vi "Do.vi"(8 "error in (no error)":errorcluster, 10 "Actor in":refnum<class "Actor.lvclass">, 11 "Configure Ports Msg":refnum<class "Configure Ports Msg.lvclass">) -> (0 "error out":errorcluster, 2 "Actor out":refnum<class "Actor.lvclass">)   [LabVIEW 2015, in "Generic Data Acquisition.lvlib" / "National Instrument USB-6501.lvlib" / "Configure Ports Msg.lvclass"]
doc: "This VI delivers the message to the actor by calling the appropriate method(s) on the actor."
uses:
  Configure Ports Msg.lvclass
  <vilib>/ActorFramework/Actor/Actor.lvclass
  National Instrument USB-6501/National Instrument USB-6501.lvclass
  Configure Ports Msg.lvclass/Configure Ports Msg.ctl
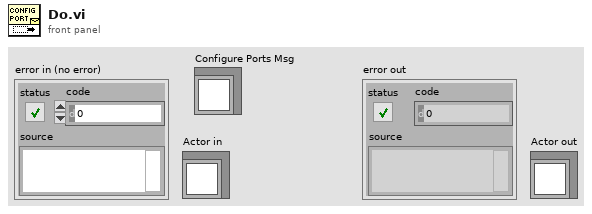
[diagram p1: front panel]
types:
  T1 = typedef "Data Acquisition Channel Settings.ctl" = cluster{"Function":enum16{"Digital Input", "Digital Output"}, "Port":i8, "Line":i8, "Name":string}
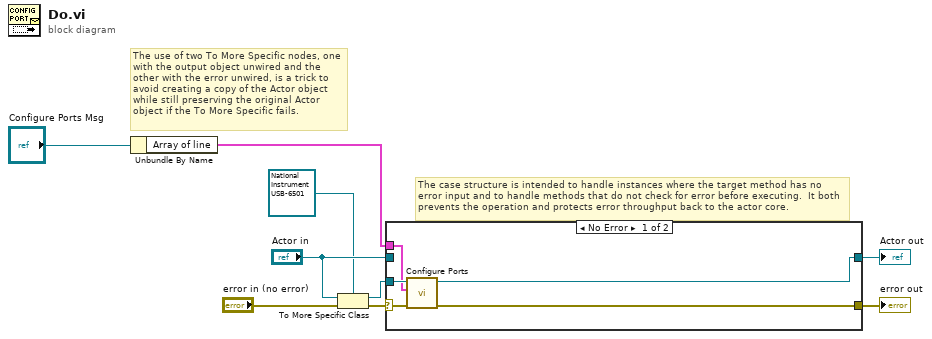
[diagram p0: block diagram]
diagram:
  # "The use of two To More Specific nodes, one with the output object unwired and the other with the error unwired, is a trick to avoid creating a copy of the Actor object while still preserving the original Actor object if the To More Specific fails."
  # "The case structure is intended to handle instances where the target method has no error input and to handle methods that do not check for error before executing.  It both prevents the operation and protects error throughput back to the actor core."
  n1 = Unbundle By Name("Configure Ports Msg") -> ("Array of line"=w3:T1[])
  n2 = To More Specific Class(target class=refnum<class "National Instrument USB-6501.lvclass"> refnum ("Generic Data Acquisition.lvlib:National Instrument USB-6501.lvlib:National Instrument USB-6501.lvclass"), reference="Actor in", error in="error in (no error)") -> (specific class reference=w2:refnum<class "National Instrument USB-6501.lvclass">, error out=w8:errorcluster)
  n3 = case shown="No Error" w8 {
    selector: w8 -> [w12 w16]
    tunnel: [w11 w16] -> w7
    tunnel: [w10 w15] -> w6
    tunnel: "Actor in" -> [_ w15]
    tunnel: w3 -> [w13 _]
    tunnel: w2 -> [w14 _]
    frame No Error {
      n4 = call-dynamic "Configure Ports.vi"("error in (no error)"=w12, "Array of line"=w13, "National Instrument USB-6501 in"=w14) -> ("error out"=w11:errorcluster, "National Instrument USB-6501 out"=w10:refnum<class "National Instrument USB-6501.lvclass">)  [unwired: 7 in]
    }
    frame Error {
    }
  }
  "error out" <- w7
  "Actor out" <- w6
